vi "Inst.KH7008.Open.vi"(8 "error in (no error)":errorcluster, 9 "index":i32=1 min=1, 10 "address":string, 11 "Inst.Krohn-Hite-7008 in":refnum<class "Inst.Krohn-Hite-7008.lvclass">) -> (0 "error out":errorcluster, 3 "Inst.Krohn-Hite-7008 out":refnum<class "Inst.Krohn-Hite-7008.lvclass">)   [LabVIEW 2019, in "Inst.KH7008.lvlib" / "Inst.Krohn-Hite-7008.lvclass"]
doc: "Use if you need to address multiple Krohn-Hite amplifiers attached to a single computer\n\n<b>index</b> is <b>1</b> for the first amplifier, etc\n\n<b>address</b> is used to access an amplifier attached to computer other than local."
uses:
  Inst.Krohn-Hite-7008.lvclass
  Inst.Krohn-Hite-7008.lvclass/Inst.Krohn-Hite-7008.ctl
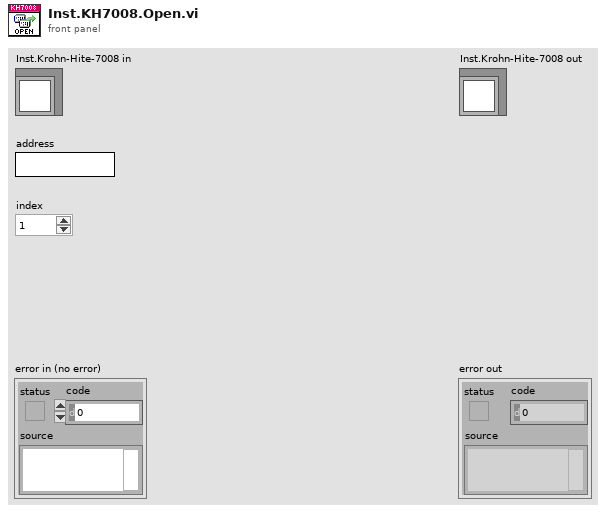
[diagram p1: front panel]
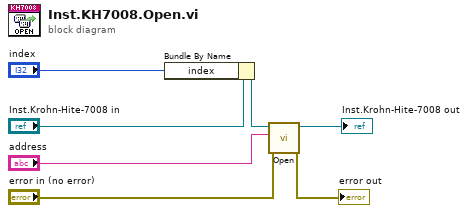
[diagram p0: block diagram]
diagram:
  n1 = Bundle By Name(cluster="Inst.Krohn-Hite-7008 in", "index"="index") -> (w2:refnum<class "Inst.Krohn-Hite-7008.lvclass">)
  n2 = call-dynamic "Open.vi"("error in (no error)"="error in (no error)", "address"="address", "Inst.Krohn-Hite-7008 in"=w2) -> ("error out"=→"error out":errorcluster, "Inst.Krohn-Hite-7008 out"=→"Inst.Krohn-Hite-7008 out":refnum<class "Inst.Krohn-Hite-7008.lvclass">)  [unwired: 7 in]
